vi "GetRoomReportData.vi"(8 "error in":errorcluster, 9 "From":timestamp, 10 "To":timestamp, 11 "Rooms":string[](array[string])) -> (0 "error out":errorcluster, 2 "RoomReport":T1)   [LabVIEW 2015]
uses:
  TypeDef/RoomReport.ctl
  Database/DatabaseApi.lvlib
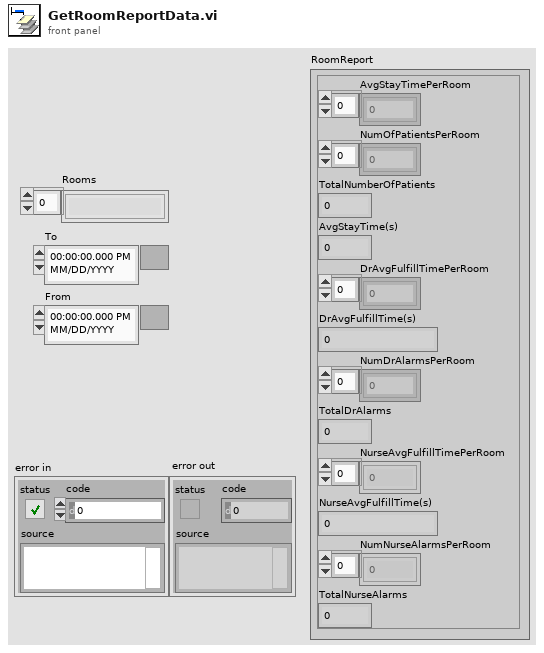
[diagram p1: front panel]
types:
  T1 = typedef "RoomReport.ctl" = cluster{"AvgStayTimePerRoom":dbl[], "NumOfPatientsPerRoom":i32[], "TotalNumberOfPatients":i32, "AvgStayTime(s)":dbl, "DrAvgFulfillTimePerRoom":dbl[], "DrAvgFulfillTime(s)":dbl, "NumDrAlarmsPerRoom":i32[], "TotalDrAlarms":i32, "NurseAvgFulfillTimePerRoom":dbl[], "NurseAvgFulfillTime(s)":dbl, "NumNurseAlarmsPerRoom":i32[], "TotalNurseAlarms":i32}
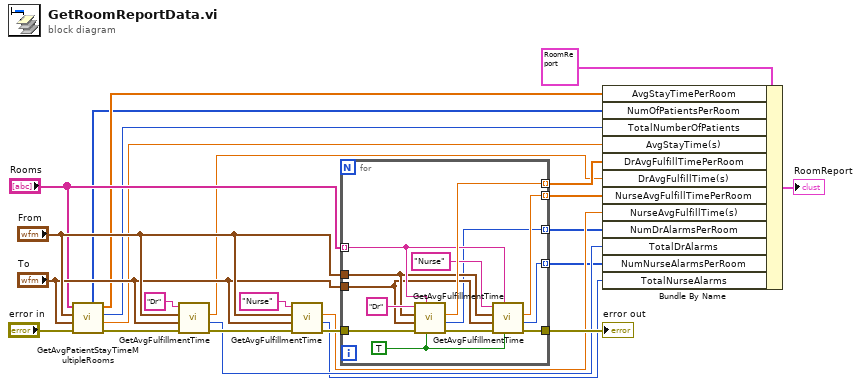
[diagram p0: block diagram]
diagram:
  n1 = call "GetAvgPatientStayTimeMultipleRooms.vi"("error in"="error in", "To"="To", "From"="From", "Rooms"="Rooms") -> ("error out"=w23:errorcluster, "AvgStayTime(s)"=w9:dbl, "TotalNumberOfPatients"=w10:i32, "AvgStayTimePerRoom"=w12:dbl[], "NumOfPatientsPerRoom"=w11:i32[])  [unwired: 3 in]
  n2 = call "GetAvgFulfillmentTime.vi"("error in"=w23, "To"="To", "From"="From", "PersonnelType"="Dr") -> ("error out"=w22:errorcluster, "NumOfAlarms"=w3:i32, "AvgFulfillTime(s)"=w6:dbl)  [unwired: 5 in]
  n3 = call "GetAvgFulfillmentTime.vi"("error in"=w22, "To"="To", "From"="From", "PersonnelType"="Nurse") -> ("error out"=w18:errorcluster, "NumOfAlarms"=w1:i32, "AvgFulfillTime(s)"=w5:dbl)  [unwired: 5 in]
  n4 = for {
    tunnel: [w33] -> w19
    tunnel: w18 -> [w37]
    tunnel: "From" -> [w30]
    tunnel: "To" -> [w29]
    tunnel: "Rooms" -> [w31] mode=indexing
    tunnel: [w34] -> w8 mode=indexing
    tunnel: [w27] -> w7 mode=indexing
    tunnel: [w26] -> w4 mode=indexing
    tunnel: [w25] -> w2 mode=indexing
    w28 = TRUE ("EnableRoomFilter")
    n5 = call "GetAvgFulfillmentTime.vi"("EnableRoomFilter"=w28, "RoomNumber"=w31, "error in"=w37, "To"=w29, "From"=w30, "PersonnelType"="Dr") -> ("error out"=w36:errorcluster, "NumOfAlarms"=w26:i32, "AvgFulfillTime(s)"=w34:dbl)  [unwired: 3 in]
    n6 = call "GetAvgFulfillmentTime.vi"("EnableRoomFilter"=w28, "RoomNumber"=w31, "error in"=w36, "To"=w29, "From"=w30, "PersonnelType"="Nurse") -> ("error out"=w33:errorcluster, "NumOfAlarms"=w25:i32, "AvgFulfillTime(s)"=w27:dbl)  [unwired: 3 in]
  }
  "error out" <- w19
  n7 = Bundle By Name(cluster=T1 {"AvgStayTimePerRoom"=[], "NumOfPatientsPerRoom"=[], "TotalNumberOfPatients"=0, "AvgStayTime(s)"=0.0, "DrAvgFulfillTimePerRoom"=[], "DrAvgFulfillTime(s)"=0.0, "NumDrAlarmsPerRoom"=[], "TotalDrAlarms"=0, "NurseAvgFulfillTimePerRoom"=[], "NurseAvgFulfillTime(s)"=0.0, "NumNurseAlarmsPerRoom"=[], "TotalNurseAlarms"=0} ("RoomReport"), "AvgStayTimePerRoom"=w12, "NumOfPatientsPerRoom"=w11, "TotalNumberOfPatients"=w10, "AvgStayTime(s)"=w9, "DrAvgFulfillTimePerRoom"=w8, "DrAvgFulfillTime(s)"=w6, "NurseAvgFulfillTimePerRoom"=w7, "NurseAvgFulfillTime(s)"=w5, "NumDrAlarmsPerRoom"=w4, "TotalDrAlarms"=w3, "NumNurseAlarmsPerRoom"=w2, "TotalNurseAlarms"=w1) -> (→"RoomReport":T1)
